vi "From Datum.vi"(0 "Value":refnum<class "Datum.lvclass">, 1 "Key":string) -> (2 "Map":refnum<class "Map.lvclass">)   [LabVIEW 2018, in "Toolkit.lvlib" / "Data.lvlib" / "Map.lvclass"]
uses:
  Map.lvclass
  Datum/Datum.lvclass
  Map.lvclass/Map.ctl
  Pair/Pair.lvclass
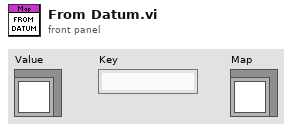
[diagram p1: front panel]
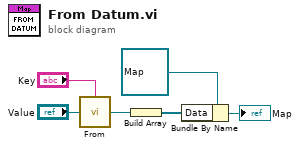
[diagram p0: block diagram]
diagram:
  n1 = call-poly "From.vi"("Value"="Value", "Key"="Key") -> ("Pair"=w1:refnum<class "Pair.lvclass">)
  n2 = Build Array(w1) -> (w4:refnum<class "Pair.lvclass">[])
  n3 = Bundle By Name(cluster=refnum<class "Map.lvclass"> refnum ("Toolkit.lvlib:Data.lvlib:Map.lvclass"), "Data"=w4) -> (→"Map":refnum<class "Map.lvclass">)
